vi "Lipgap Front View 2.vi"(0 "Image Out":T7(plugin-control), 1 "ROI Descriptor":T1 {"Contours"."Type" items=["No Selection", "Point", "Line", "Rectangle", "Oval", "Polygon", "Free", "Annulus", "Unused2", "Unused3", "Broken Line", "Free Hand Line", "Rotated Rectangle"]}, 2 "Edge Options":T3={"Edge Polarity"=2, "Kernel Size"=3, "Width"=3, "Minimum Edge Strength"=50.0, "Interpolation Type"=enum."Zero Order", "Data Processing Method"=enum."Average"} {"Edge Polarity" items=["All Edges", "Rising Edges", "Falling Edges"]; "Minimum Edge Strength" format="%.2f"; "Width" step=2; "Kernel Size" step=2}, 3 "Line Options":T5={"Number of Lines"=1, "Type"=enum."Best Edge Rake", "Min. Score"=10.0, "Max. Score"=1000.0, "Orientation"=0.0, "Angle Range"=70.0, "Angle Tolerance"=1.0, "Step Size"=12, "Min. SNR (db)"=0.0, "Min. Points (%)"=25.0, "Hough Iterations"=5} {"Min. Points (%)" min=0.0 max=100.0; "Min. SNR (db)" min=0.0; "Max. Score" min=0.0 max=1024.0; "Min. Score" min=0.0 max=1024.0 step=1.0}, 5 "error in (no error)":errorcluster) -> (14 "x/y":sgl, 15 "mm value":sgl, 19 "error out":errorcluster)   [LabVIEW 2015]
uses:
  <vilib>/vision/Measure.llb/Straight Edge Options.ctl
  <vilib>/vision/Measure.llb/Straight Edge Process.ctl
  <vilib>/vision/Measure.llb/Edge Options.ctl
  <vilib>/vision/Measure.llb/Edge Polarity.ctl
  <vilib>/vision/Measure.llb/Edge New.ctl
  <vilib>/vision/NI_Vision_Development_Module.lvlib
  FrameworkOverrides/Algorithm.lvclass
panel:
  out "Array 3":sgl[](array[numeric])
  out "Edge Information 2":T2[][](array[typedef]) {"Distance (Real-World)" format="%.2f"; "Location (Real-World)"."Y" format="%.2g"; "Location (Real-World)"."X" format="%.2f"; "Noise" format="%.2f"; "Location (Pixel)"."Y" format="%.2g"; "Location (Pixel)"."X" format="%.2f"; "Strength" format="%.2f"; "Distance (Pixel)" format="%.2f"}
  out "Edge Information":T2[][](array[typedef]) {"Distance (Real-World)" format="%.2f"; "Location (Real-World)"."Y" format="%.2g"; "Location (Real-World)"."X" format="%.2f"; "Noise" format="%.2f"; "Location (Pixel)"."Y" format="%.2g"; "Location (Pixel)"."X" format="%.2f"; "Strength" format="%.2f"; "Distance (Pixel)" format="%.2f"}
  in  "Y_offset_Bottom":i32=85
  in  "Y_offset_Top":i32=98
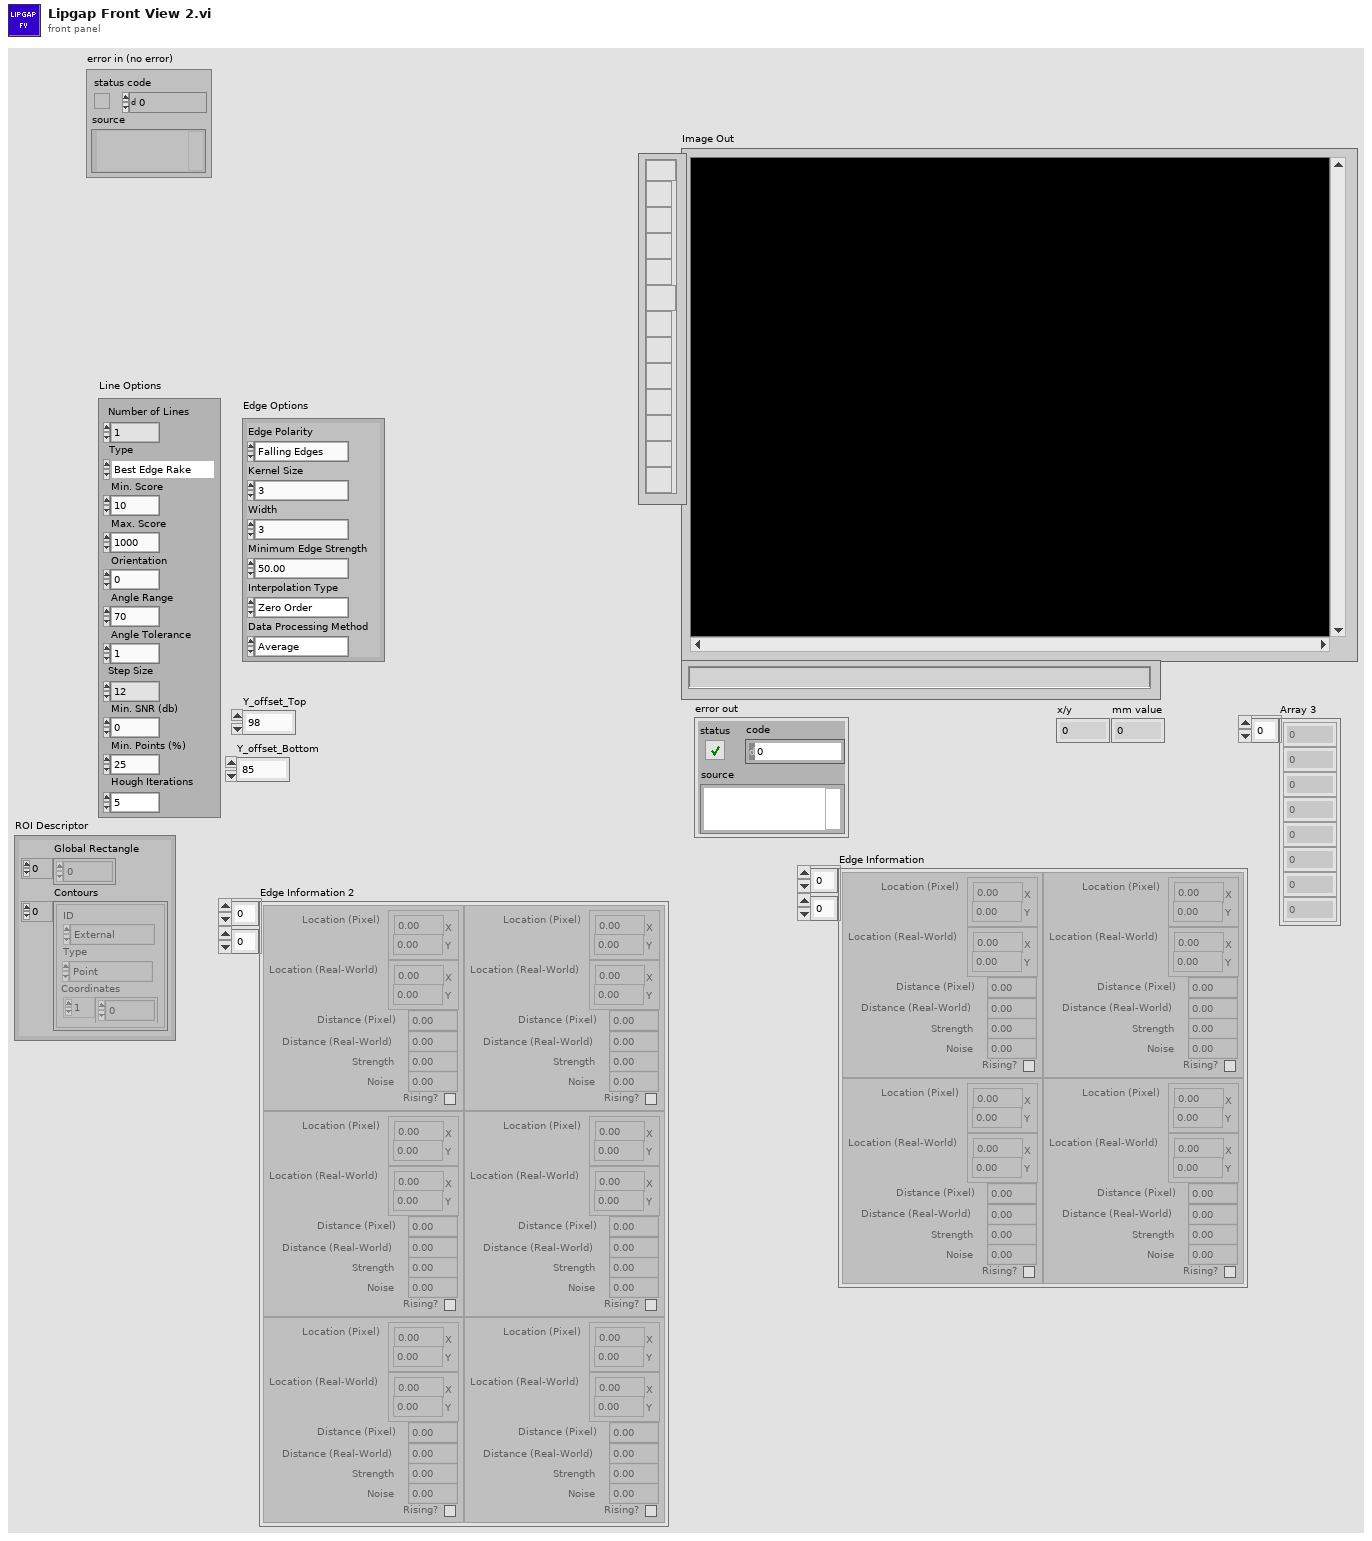
[diagram p1: front panel]
types:
  T1 = cluster{"Global Rectangle":i32[], "Contours":cluster{"ID":enum32{"External", "Internal"}, "Type":u32, "Coordinates":i32[]}[]}
  T2 = typedef "Edge New.ctl" = cluster{"Location (Pixel)":cluster{"X":sgl, "Y":sgl}, "Location (Real-World)":cluster{"X":sgl, "Y":sgl}, "Distance (Pixel)":dbl, "Distance (Real-World)":dbl, "Strength":dbl, "Noise":dbl, "Rising?":bool}
  T3 = typedef "Edge Options.ctl" = cluster{"Edge Polarity":T4, "Kernel Size":u32, "Width":u32, "Minimum Edge Strength":sgl, "Interpolation Type":enum32{"Zero Order", "Bilinear", "Quadratic", "Cubic", "Bilinear Fixed"}, "Data Processing Method":enum32{"Average", "Median"}}
  T4 = typedef "Edge Polarity.ctl" = u32
  T5 = typedef "Straight Edge Options.ctl" = cluster{"Number of Lines":i32, "Type":T6, "Min. Score":dbl, "Max. Score":dbl, "Orientation":dbl, "Angle Range":dbl, "Angle Tolerance":dbl, "Step Size":u32, "Min. SNR (db)":dbl, "Min. Points (%)":dbl, "Hough Iterations":i32}
  T6 = typedef "Straight Edge Process.ctl" = enum32{"First Edge Rake", "Best Edge Rake", "Hough Edge Rake", "First Edge Projection", "Best Edge Projection"}
  T7 = typedef "IMAQ Image.ctl" = refnum<image>
  T8 = enum16{"Get First Edge", "Get First + Last Edge", "Get All Edges", "Get Best Edge"}
  T9 = typedef "IMAQ Rectangle" = cluster{"Left":i32, "Top":i32, "Right":i32, "Bottom":i32, "Rotation":dbl}
  T10 = cluster{"Point1 (Pixels)":cluster{"X":sgl, "Y":sgl}, "Point2 (Pixels)":cluster{"X":sgl, "Y":sgl}, "Point1 (Real-World)":cluster{"X":sgl, "Y":sgl}, "Point2 (Real-World)":cluster{"X":sgl, "Y":sgl}, "Angle (Pixel)":dbl, "Angle (Real-World)":dbl, "Score":dbl, "Straightness":dbl, "Average SNR (db)":dbl, "Calibration Valid":bool}[]
  T11 = cluster{"Point1 (Pixels)":cluster{"X":sgl, "Y":sgl}, "Point2 (Pixels)":cluster{"X":sgl, "Y":sgl}, "Point1 (Real-World)":cluster{"X":sgl, "Y":sgl}, "Point2 (Real-World)":cluster{"X":sgl, "Y":sgl}, "Angle (Pixel)":dbl, "Angle (Real-World)":dbl, "Score":dbl, "Straightness":dbl, "Average SNR (db)":dbl, "Calibration Valid":bool}
  T12 = typedef "ROI Descriptor" = cluster{"Global Rectangle":i32[], "Contours":cluster{"ID":enum32{"External", "Internal"}, "Type":u32, "Coordinates":i32[]}[]}
  T13 = typedef "Search Line.ctl" = cluster{"Start Point":cluster{"X":sgl, "Y":sgl}, "End Point":cluster{"X":sgl, "Y":sgl}, "Edge Info":T2[], "Edge Map":dbl[], "Calibration Valid":bool}
  T14 = typedef "IMAQ Line" = cluster{"Start X":i32, "Start Y":i32, "End X":i32, "End Y":i32}
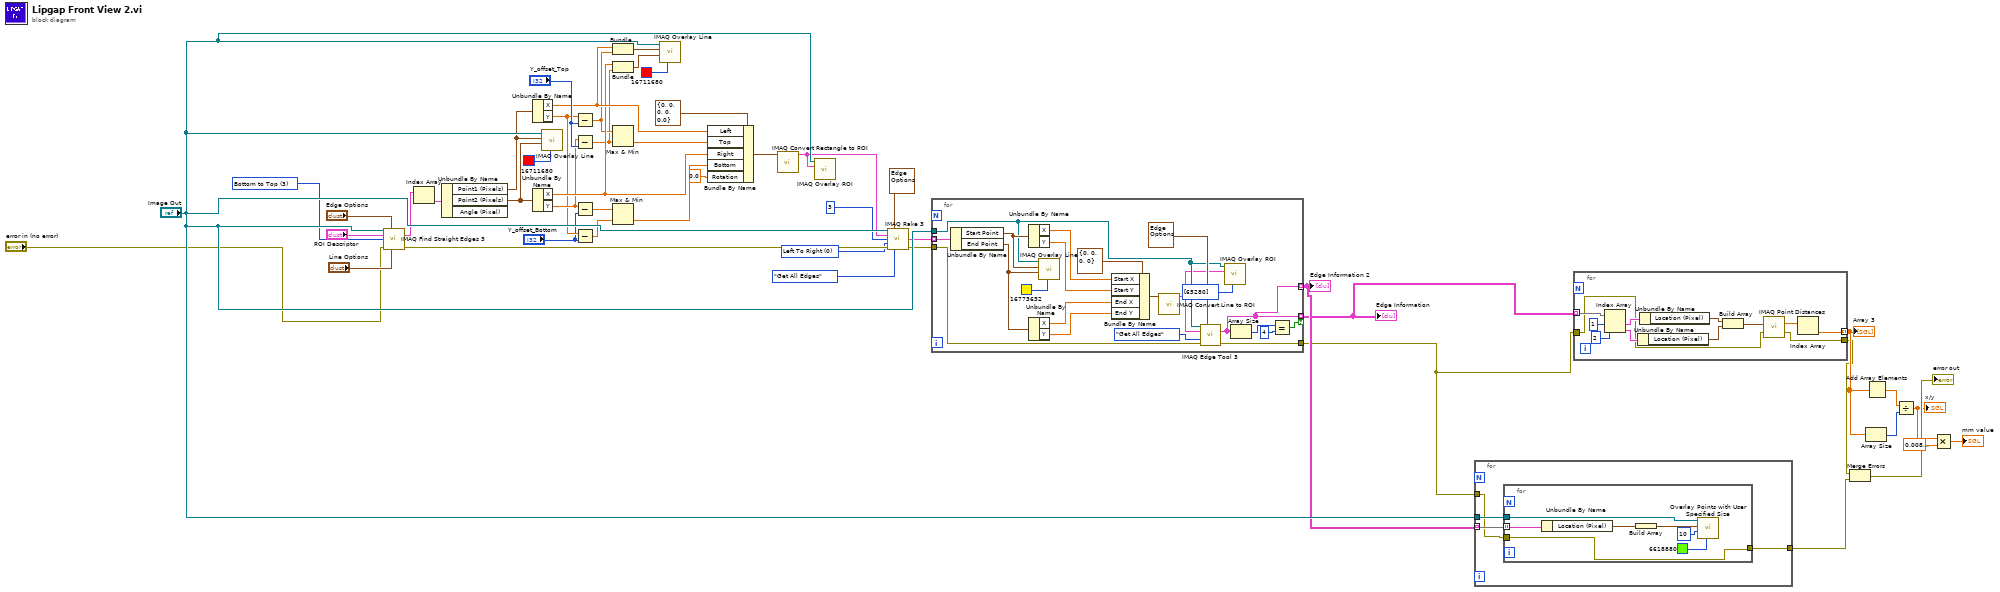
[diagram p0: block diagram]
diagram:
  w48 = u32 3 items=["Left to Right", "Right to Left", "Top to Bottom", "Bottom to Top"] ("Search Direction")
  w18 = u16 0 items=["Left To Right", "Right To Left", "Top To Bottom", "Bottom To Top"] ("Scan Direction")
  n1 = call "IMAQ Find Straight Edges 3"("Image"="Image Out", "Edge Options"="Edge Options", "ROI Descriptor"="ROI Descriptor", "Search Direction"=w48, "error in (no error)"="error in (no error)", "Line Options"="Line Options") -> ("Straight Edges"=w45:T10, "error out"=w23:errorcluster)  [unwired: 5 in, 3 out]
  n2 = Index Array(array=w45) -> (element=w44:T11)  [unwired: 1 in]
  n3 = Unbundle By Name(w44) -> ("Point1 (Pixels)"=w42:cluster{"X":sgl, "Y":sgl}, "Point2 (Pixels)"=w41:cluster{"X":sgl, "Y":sgl})  [unwired: 1 out]
  n4 = Unbundle By Name(w42) -> ("X"=w35:sgl, "Y"=w31:sgl)
  n5 = Unbundle By Name(w41) -> ("X"=w34:sgl, "Y"=w32:sgl)
  n6 = call "IMAQ Overlay Line"("Color"=u32 16711680, "End Point"=w41, "Start Point"=w42, "Image"="Image Out") -> ()  [unwired: 6 in, 2 out]
  n7 = Subtract(x=w31, y="Y_offset_Top") -> (x-y=w25:sgl)
  n8 = Subtract(x=w32, y="Y_offset_Top") -> (x-y=w24:sgl)
  n9 = Subtract(x=w32, y="Y_offset_Bottom") -> (x-y=w29:sgl)
  n10 = Subtract(x=w31, y="Y_offset_Bottom") -> (x-y=w28:sgl)
  n11 = Bundle("X"=w35, w25) -> (w38:cluster{"X":sgl, sgl})  [unwired: 1 in]
  n12 = Bundle("X"=w34, w24) -> (w37:cluster{"X":sgl, sgl})  [unwired: 1 in]
  n13 = Max & Min(x=w25, y=w24) -> (min(x,y)=w33:sgl)  [unwired: 1 out]
  n14 = Max & Min(x=w29, y=w28) -> (min(x,y)=w26:sgl)  [unwired: 1 out]
  n15 = call "IMAQ Overlay Line"("Color"=u32 16711680, "End Point"=w37, "Start Point"=w38, "Image"="Image Out") -> ()  [unwired: 6 in, 2 out]
  n16 = Bundle By Name(cluster=T9 {"Left"=0, "Top"=0, "Right"=0, "Bottom"=0, "Rotation"=0.0} ("Rectangle"), "Left"=w35, "Top"=w33, "Right"=w34, "Bottom"=w26, "Rotation"=0.0) -> (w27:T9)
  n17 = call "IMAQ Convert Rectangle to ROI"("Rectangle"=w27) -> ("ROI Descriptor"=w22:T12)  [unwired: 8 in, 1 out]
  n18 = call "IMAQ Overlay ROI"("ROI Descriptor"=w22, "Image"="Image Out") -> ()  [unwired: 8 in, 2 out]
  n19 = call "IMAQ Rake 3"("Image"="Image Out", "Edge Options"=T3 {"Edge Polarity"=0, "Kernel Size"=3, "Width"=3, "Minimum Edge Strength"=50.0, "Interpolation Type"=enum."Zero Order", "Data Processing Method"=enum."Average"} ("Edge Options 2"), "ROI Descriptor"=w22, "Step Size"=u32 3, "Scan Direction"=w18, "error in (no error)"=w23, "Process"=T8."Get All Edges") -> ("Search Lines"=w16:T13[], "error out"=w15:errorcluster)  [unwired: 5 in, 2 out]
  n20 = for {
    tunnel: w16 -> [w70] mode=indexing
    tunnel: "Image Out" -> [w52]
    tunnel: [w53] -> w13 mode=indexing if=w56
    tunnel: w15 -> [w55]
    tunnel: [w54] -> w8
    tunnel: [w53] -> w14 mode=indexing
    n21 = Unbundle By Name(w70) -> ("Start Point"=w67:cluster{"X":sgl, "Y":sgl}, "End Point"=w65:cluster{"X":sgl, "Y":sgl})
    n22 = Unbundle By Name(w67) -> ("X"=w63:sgl, "Y"=w62:sgl)
    n23 = Unbundle By Name(w65) -> ("X"=w66:sgl, "Y"=w64:sgl)
    n24 = call "IMAQ Overlay Line"("Color"=u32 16773632, "End Point"=w65, "Start Point"=w67, "Image"=w52) -> ()  [unwired: 6 in, 2 out]
    n25 = Bundle By Name(cluster=T14 {"Start X"=0, "Start Y"=0, "End X"=0, "End Y"=0} ("Line"), "Start X"=w63, "Start Y"=w62, "End X"=w66, "End Y"=w64) -> (w61:T14)
    n26 = call "IMAQ Convert Line to ROI"("Line"=w61) -> ("ROI Descriptor"=w51:T12)  [unwired: 8 in, 1 out]
    n27 = call "IMAQ Edge Tool 3"("Image"=w52, "Edge Options"=T3 {"Edge Polarity"=0, "Kernel Size"=3, "Width"=3, "Minimum Edge Strength"=50.0, "Interpolation Type"=enum."Bilinear Fixed", "Data Processing Method"=enum."Average"} ("Edge Options 3"), "ROI Descriptor"=w51, "Process"=T8."Get All Edges", "error in (no error)"=w55) -> ("Edge Information"=w53:T2[], "error out"=w54:errorcluster)  [unwired: 6 in, 3 out]
    n28 = call "IMAQ Overlay ROI"("Colors (Green)"=u32[] [65280], "ROI Descriptor"=w51, "Image"=w52) -> ()  [unwired: 7 in, 2 out]
    n29 = Array Size(array=w53) -> (size(s)=w58:i32)
    n30 = Equal?(x=w58, y=4) -> (x = y?=w56:bool)
  }
  "Edge Information" <- w13
  "Edge Information 2" <- w14
  n31 = for {
    tunnel: w14 -> [w73] mode=indexing
    tunnel: "Image Out" -> [w74]
    tunnel: w8 -> [w72]
    tunnel: [w71] -> w9
    n32 = for {
      tunnel: w74 -> [w81]
      tunnel: w73 -> [w80] mode=indexing
      tunnel: w72 -> [w75]
      tunnel: [w75] -> w71
      n33 = Unbundle By Name(w80) -> ("Location (Pixel)"=w79:cluster{"X":sgl, "Y":sgl})
      n34 = Build Array(w79) -> (w78:cluster{"X":sgl, "Y":sgl}[])
      n35 = call "Overlay Points with User Specified Size.vi"("Color"=u32 6618880, "Point Diameter (5)"=u32 10, "Points"=w78, "Image In"=w81) -> ()  [unwired: 6 in, 2 out]
    }
  }
  n36 = for {
    tunnel: w13 -> [w93] mode=indexing
    tunnel: [w87] -> w12 mode=indexing
    tunnel: w8 -> [w83]
    tunnel: [w82] -> w7
    n37 = Index Array(array=w93, index #1=1 ("index"), index #2=2 ("index")) -> (element #1=w92:T2, element #2=w91:T2)
    n38 = Unbundle By Name(w91) -> ("Location (Pixel)"=w85:cluster{"X":sgl, "Y":sgl})
    n39 = Unbundle By Name(w92) -> ("Location (Pixel)"=w86:cluster{"X":sgl, "Y":sgl})
    n40 = Build Array(w86, w85) -> (w84:cluster{"X":sgl, "Y":sgl}[])
    n41 = call "IMAQ Point Distances"("Points"=w84, "error in (no error)"=w83) -> ("Distances"=w88:sgl[], "error out"=w82:errorcluster)  [unwired: 3 in]
    n42 = Index Array(array=w88) -> (element=w87:sgl)  [unwired: 1 in]
  }
  "Array 3" <- w12
  n43 = Merge Errors(w7, w9) -> (→"error out":errorcluster)
  n44 = Array Size(array=w12) -> (size(s)=w10:i32)
  n45 = Add Array Elements(numeric array=w12) -> (sum=w11:sgl)
  n46 = Divide(x=w11, y=w10) -> (x/y=w3:sgl)
  "x/y" <- w3
  n47 = Multiply(x=w3, y=sgl 0.009) -> (x*y=→"mm value":sgl)
